vi "Initialize LogEngine Events.vi"(8 "error in (no error)":errorcluster, 11 "LogEngine.lvclass":refnum<class "LogEngine.lvclass">) -> (0 "error out":errorcluster, 3 "LogEngine.lvclass":refnum<class "LogEngine.lvclass">)   [LabVIEW 2017, in "LogEngine.lvclass"]
doc: "Developed by Kevin Thompson\nkevin@thompsonengineering.net\n\nCopyright 2018-2020\nThompson Engineering, LLC"
uses:
  LogEngine.lvclass
  Data Types/TD LoggerStateChanged EventData--cluster.ctl
  Data Types/TD Logger State Data--cluster.ctl
  Data Types/TD Logger State--enum.ctl
  Ichor_Common/DataTypes/TD Async CmdMsg EventData--cluster.ctl
  LogEngine.lvclass/LogEngine.ctl
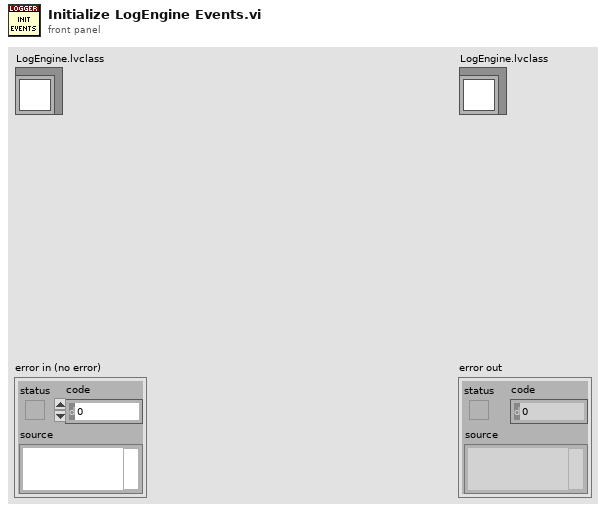
[diagram p1: front panel]
types:
  T1 = typedef "LogEngine.lvclass/TD LoggerStateChanged EventData--cluster.ctl" = cluster{"Time Stamp":timestamp, "OLD State Data":T2, "NEW State Data":T2}
  T2 = typedef "LogEngine.lvclass/TD Logger State Data--cluster.ctl" = cluster{"Logger State":T3, "TDMS Logging State":T3, "LogFile path":path, "TDMS File path":path, "vData":variant}
  T3 = typedef "LogEngine.lvclass/TD Logger State--enum.ctl" = enum16{"Unknown", "Logging", "NotLogging", "Error"}
  T4 = typedef "TD Async CmdMsg EventData--cluster.ctl" = cluster{"Time Stamp":timestamp, "CmdMsg":string, "vData":variant}
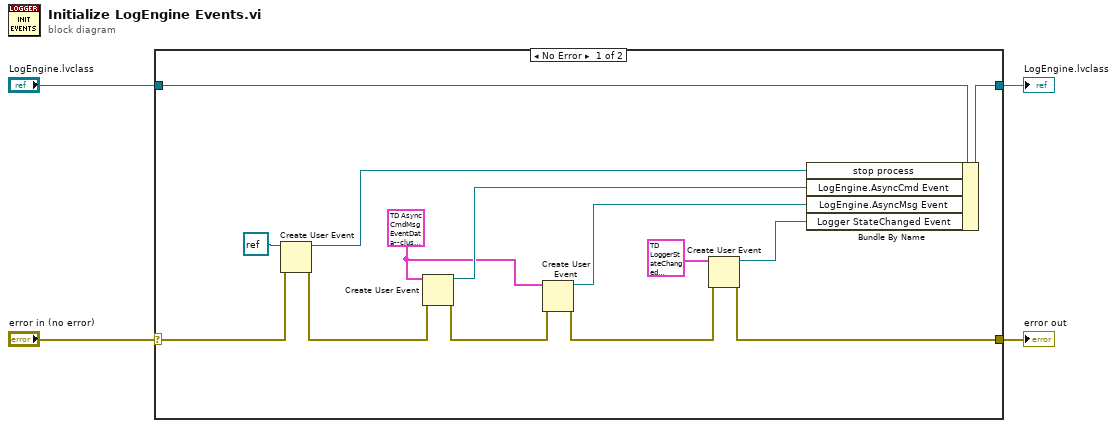
[diagram p0: block diagram]
diagram:
  n1 = case shown="No Error" "error in (no error)" {
    selector: "error in (no error)" -> [w9 w20]
    tunnel: [w12 w20] -> w3
    tunnel: [w17 w19] -> w1
    tunnel: "LogEngine.lvclass" -> [w18 w19]
    frame No Error {
      w6 = T4 {"Time Stamp"=timestamp(0 s since 1904-01-01), "CmdMsg"="", "vData"=variant} ("Async EvData")
      n2 = Create User Event(user event datatype=refnum<notifier> refnum ("notifier out"), error in=w9) -> (user event=w15:refnum<user-event>, error out=w14:errorcluster)
      n3 = Create User Event(user event datatype=w6, error in=w14) -> (user event=w13:refnum<user-event>, error out=w8:errorcluster)
      n4 = Create User Event(user event datatype=w6, error in=w8) -> (user event=w5:refnum<user-event>, error out=w7:errorcluster)
      n5 = Create User Event(user event datatype=T1 {"Time Stamp"=timestamp(0 s since 1904-01-01), "OLD State Data"={"Logger State"=enum."Logging", "TDMS Logging State"=enum."Unknown", "LogFile path"=path "", "TDMS File path"=path "", "vData"=variant}, "NEW State Data"={"Logger State"=enum."Logging", "TDMS Logging State"=enum."Unknown", "LogFile path"=path "", "TDMS File path"=path "", "vData"=variant}} ("DAQStateChanged EventData"), error in=w7) -> (user event=w10:refnum<user-event>, error out=w12:errorcluster)
      n6 = Bundle By Name(cluster=w18, "stop process"=w15, "LogEngine.AsyncCmd Event"=w13, "LogEngine.AsyncMsg Event"=w5, "Logger StateChanged Event"=w10) -> (w17:refnum<class "LogEngine.lvclass">)
    }
    frame Error {
    }
  }
  "error out" <- w3
  "LogEngine.lvclass" <- w1
